vi "Launch Python Connector.vi"(7 "Path to python.exe":path, 8 "error in (no error)":errorcluster, 9 "Ports":T1={"KA Port (9007)"=9007, "LtoP Port (9008)"=9008, "PtoL Port (9009)"=9009}, 10 "Tell Python the IP Address Where LabVIEW Is":string, 11 "Path to Python Core Folder":path) -> (0 "error out":errorcluster)   [LabVIEW 2013, in "TS.lvlib"]
doc: "If we're letting LabVIEW start up TestScript, then this VI runs the Python command in Windows to start it up. Note that we pass in the argument Tell Python Where LabVIEW Is, which tells the connector automatically to use the IP address in the argument."
uses:
  TS.lvlib
  Ports - Keep-Alive, LabVIEW-to-Python, Python-to-LabVIEW.ctl
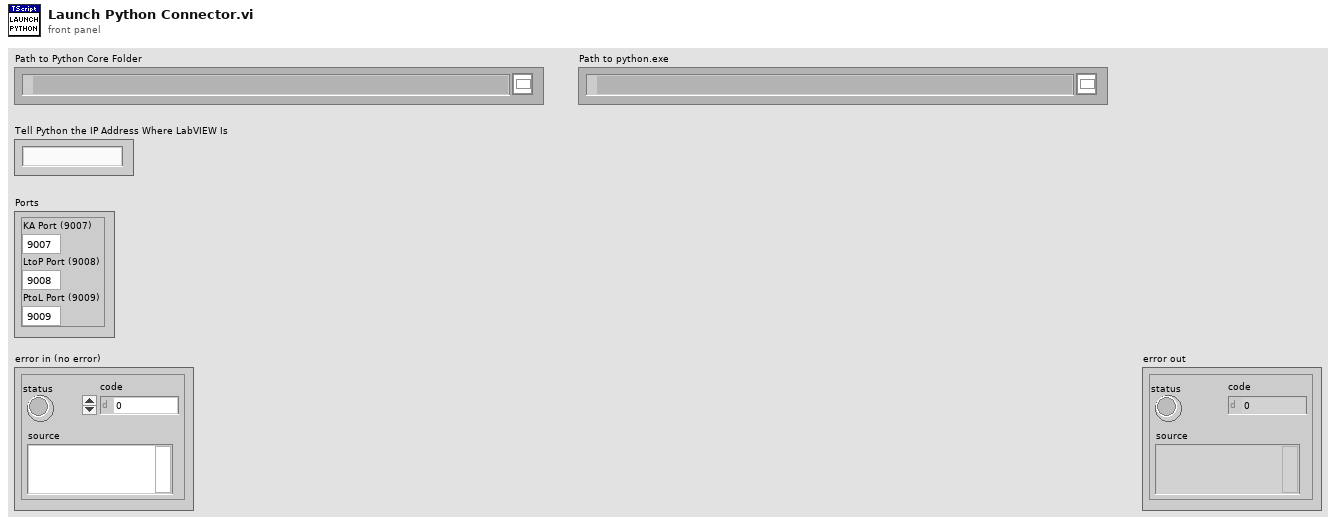
[diagram p1: front panel]
types:
  T1 = typedef "TS.lvlib/Ports - Keep-Alive, LabVIEW-to-Python, Python-to-LabVIEW.ctl" = cluster{"KA Port (9007)":u16, "LtoP Port (9008)":u16, "PtoL Port (9009)":u16}
  T2 = cluster{"KA Port (9007)":string, "LtoP Port (9008)":string, "PtoL Port (9009)":string}
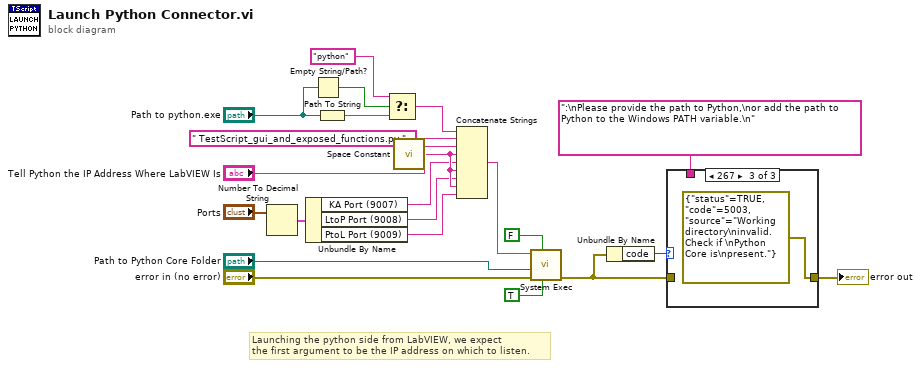
[diagram p0: block diagram]
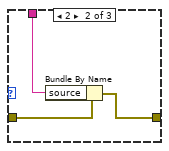
[diagram p3: hidden frame]
diagram:
  # "Launching the python side from LabVIEW, we expect \nthe first argument to be the IP address on which to listen."
  n1 = Number To Decimal String(number="Ports") -> (decimal integer string=w4:T2)  [unwired: 1 in]
  n2 = Unbundle By Name(w4) -> ("KA Port (9007)"=w3:string, "LtoP Port (9008)"=w2:string, "PtoL Port (9009)"=w1:string)
  n3 = Empty String/Path?(string/path="Path to python.exe") -> (empty?=w18:bool)
  n4 = Path To String(path="Path to python.exe") -> (string=w15:string)
  n5 = Select(t="python" ("command line"), s=w18, f=w15) -> (s? t:f=w13:string)
  n6 = call <vilib>:"Space Constant.vi"() -> ("String"=w6:string)
  n7 = Concatenate Strings(w13, " TestScript_gui_and_exposed_functions.py " ("command line"), "Tell Python the IP Address Where LabVIEW Is", w6, w3, w6, w2, w6, w1) -> (w12:string)
  n8 = call <vilib>:"System Exec.vi"("run minimized? (F)"=TRUE, "wait until completion? (T)"=FALSE, "error in (no error)"="error in (no error)", "working directory"="Path to Python Core Folder", "command line"=w12) -> ("error out"=w11:errorcluster)  [unwired: 3 in, 3 out]
  n9 = Unbundle By Name(w11) -> ("code"=w9:i32)
  n10 = case shown="267" w9 {
    tunnel: w11 -> [w23 w26 _]
    tunnel: [w23 w25 errorcluster {"status"=TRUE, "code"=5003, "source"="Working directory\ninvalid. Check if \nPython Core is\npresent."} ("error out")] -> w10
    tunnel: ":\nPlease provide the path to Python,\nor add the path to Python to the Windows PATH variable.\n" ("source") -> [_ w24 _]
    frame Default {
    }
    frame 2 {
      n11 = Bundle By Name(cluster=w26, "source"=w24) -> (w25:errorcluster)
    }
    frame 267 {
    }
  }
  "error out" <- w10
